vi "Shooter Code.vi"(10 "velocity_lower":dbl=1.0 format="%#_13g", 11 "velocity_upper":dbl=0.9 format="%#_13g") -> ()   [LabVIEW 2015]
panel:
  in  "index":dbl=1.0
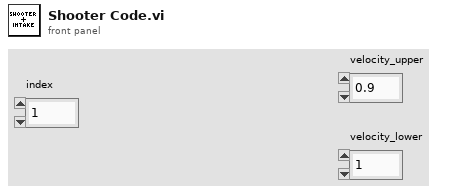
[diagram p1: front panel]
types:
  T1 = typedef "WPI_MotorControlDeviceRef.ctl" = cluster{"DeviceStatus":errorcluster, "Type":T2, "PWM":cluster{"PWM Channel":T3, "DeadBand":T4}, "CAN":cluster{"Device Number":u8, "Control Mode":T5, "Semaphore":T6, "Max Vout":dbl, "TalonSRX Control Mode":T7}, "Invert":bool}
  T2 = typedef "WPI_MotorControlType.ctl" = enum16{"PWM", "CAN", "CANTalonSRX"}
  T3 = typedef "FPGA_DIOPWMChannel.ctl" = enum8{"PWM 0", "PWM 1", "PWM 2", "PWM 3", "PWM 4", "PWM 5", "PWM 6", "PWM 7", "PWM 8", "PWM 9", "PWM MXP 0", "PWM MXP 1", "PWM MXP 2", "PWM MXP 3", "PWM MXP 4", "PWM MXP 5", "PWM MXP 6", "PWM MXP 7", "PWM MXP 8", "PWM MXP 9", "Invalid"}
  T4 = typedef "WPI_PWMDeadband.ctl" = cluster{"Name":string, "maxPositivePwm":i32, "minPositivePwm":i32, "centerPwm":i32, "maxNegativePwm":i32, "minNegativePwm":i32, "angularRange":u16}
  T5 = typedef "WPI_CANJaguar_ControlMode.ctl" = enum8{"Percent VBus", "Current", "Speed", "Position", "Voltage"}
  T6 = typedef "Semaphore RefNum" = refnum<k1>
  T7 = typedef "WPI_CANTalonSRX_APIControlMode.ctl" = enum8{"Percent VBus", "Speed", "Position", "Slave", "Unchanged / Invalid", "Voltage Compensation", "Current", "Motion Profile"}
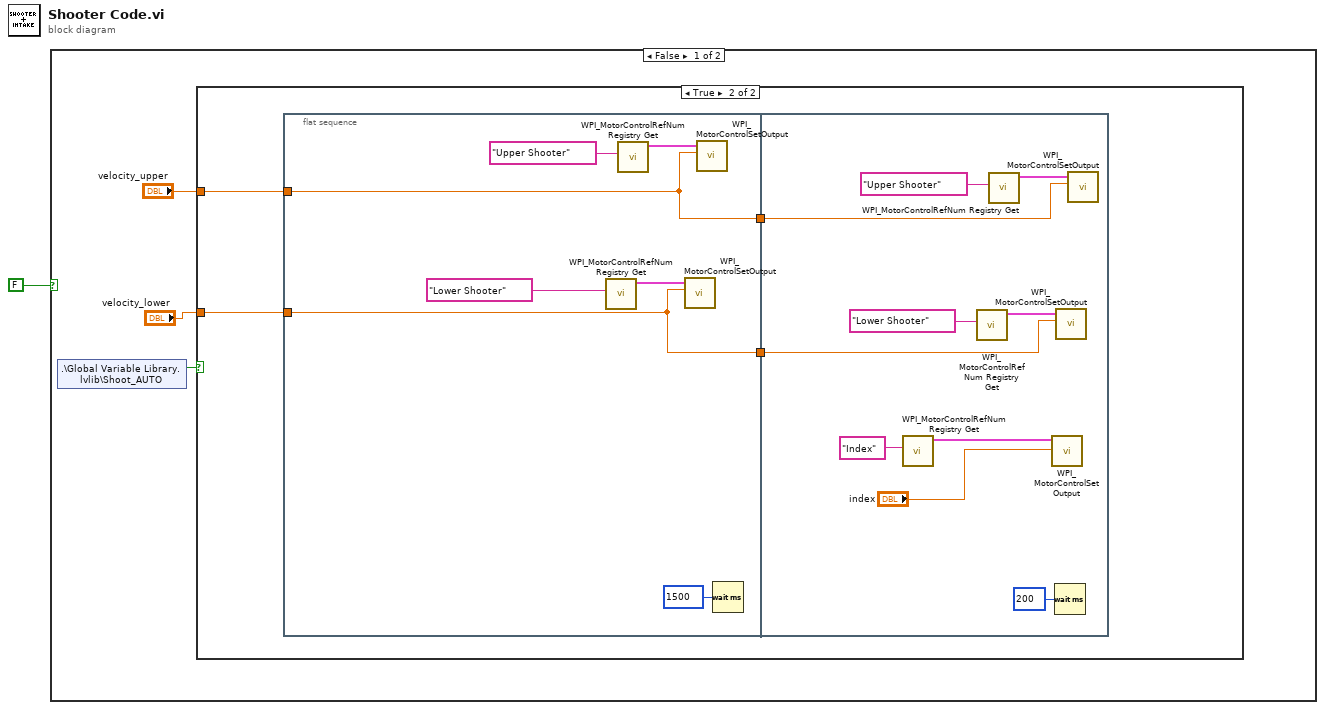
[diagram p0: block diagram]
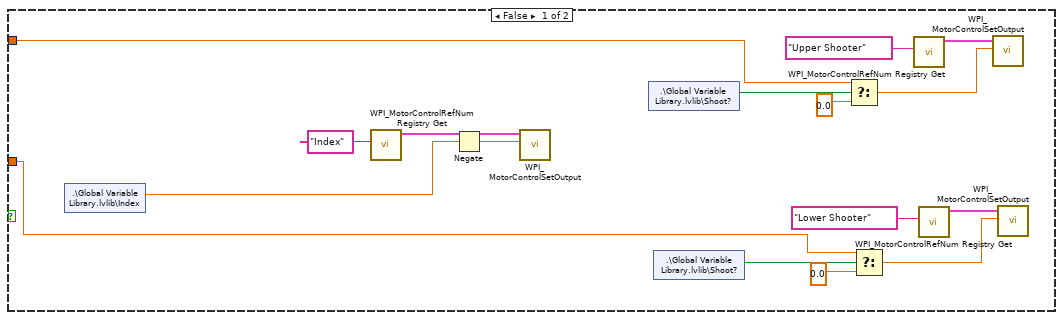
[diagram p2: hidden frame]
diagram:
  n1 = case shown="False" FALSE {
    frame False {
      n2 = shared-variable ".\\Global Variable Library.lvlib\\Shoot_AUTO"() -> (w4:bool)  [unwired: 1 in, 1 out]
      n3 = case shown="True" w4 {
        tunnel: "velocity_lower" -> [w5 w22]
        tunnel: "velocity_upper" -> [w6 w21]
        frame False {
          n4 = shared-variable ".\\Global Variable Library.lvlib\\Index"() -> (w7:dbl)  [unwired: 1 in, 1 out]
          n5 = call <vilib>:"WPI_MotorControlRefNum Registry Get.vi"("refnum name"="Index") -> ("MotorControlDevRef"=w10:T1)  [unwired: 9 in, 1 out]
          n6 = Negate(x=w7) -> (-x=w8:dbl)
          n7 = call <vilib>:"WPI_MotorControlSetOutput.vi"("Output"=w8, "MotorControlDevRef"=w10) -> ()  [unwired: 7 in, 3 out]
          n8 = shared-variable ".\\Global Variable Library.lvlib\\Shoot?"() -> (w18:bool)  [unwired: 1 in, 1 out]
          n9 = shared-variable ".\\Global Variable Library.lvlib\\Shoot?"() -> (w13:bool)  [unwired: 1 in, 1 out]
          n10 = Select(t=w6, s=w18, f=0.0) -> (s? t:f=w20:dbl)
          n11 = Select(t=w5, s=w13, f=0.0 ("f 2")) -> (s? t:f=w11:dbl)
          n12 = call <vilib>:"WPI_MotorControlRefNum Registry Get.vi"("refnum name"="Upper Shooter") -> ("MotorControlDevRef"=w16:T1)  [unwired: 9 in, 1 out]
          n13 = call <vilib>:"WPI_MotorControlRefNum Registry Get.vi"("refnum name"="Lower Shooter") -> ("MotorControlDevRef"=w15:T1)  [unwired: 9 in, 1 out]
          n14 = call <vilib>:"WPI_MotorControlSetOutput.vi"("Output"=w20, "MotorControlDevRef"=w16) -> ()  [unwired: 7 in, 3 out]
          n15 = call <vilib>:"WPI_MotorControlSetOutput.vi"("Output"=w11, "MotorControlDevRef"=w15) -> ()  [unwired: 7 in, 3 out]
        }
        frame True {
          n16 = flat-sequence {
            tunnel: [w27] -> w24
            tunnel: [w26] -> w23
            tunnel: w21 -> [w27]
            tunnel: w22 -> [w26]
            tunnel: w24 -> [w37]
            tunnel: w23 -> [w36]
            frame #0 {
              n17 = call <vilib>:"WPI_MotorControlRefNum Registry Get.vi"("refnum name"="Lower Shooter") -> ("MotorControlDevRef"=w30:T1)  [unwired: 9 in, 1 out]
              n18 = call <vilib>:"WPI_MotorControlRefNum Registry Get.vi"("refnum name"="Upper Shooter") -> ("MotorControlDevRef"=w29:T1)  [unwired: 9 in, 1 out]
              n19 = call <vilib>:"WPI_MotorControlSetOutput.vi"("Output"=w26, "MotorControlDevRef"=w30) -> ()  [unwired: 7 in, 3 out]
              n20 = call <vilib>:"WPI_MotorControlSetOutput.vi"("Output"=w27, "MotorControlDevRef"=w29) -> ()  [unwired: 7 in, 3 out]
              n21 = Wait (ms)(milliseconds to wait=u32 1500) -> ()  [unwired: 1 out]
            }
            frame #1 {
              n22 = call <vilib>:"WPI_MotorControlRefNum Registry Get.vi"("refnum name"="Index") -> ("MotorControlDevRef"=w34:T1)  [unwired: 9 in, 1 out]
              n23 = call <vilib>:"WPI_MotorControlRefNum Registry Get.vi"("refnum name"="Lower Shooter") -> ("MotorControlDevRef"=w39:T1)  [unwired: 9 in, 1 out]
              n24 = call <vilib>:"WPI_MotorControlRefNum Registry Get.vi"("refnum name"="Upper Shooter") -> ("MotorControlDevRef"=w40:T1)  [unwired: 9 in, 1 out]
              n25 = call <vilib>:"WPI_MotorControlSetOutput.vi"("Output"="index", "MotorControlDevRef"=w34) -> ()  [unwired: 7 in, 3 out]
              n26 = Wait (ms)(milliseconds to wait=u32 200) -> ()  [unwired: 1 out]
              n27 = call <vilib>:"WPI_MotorControlSetOutput.vi"("Output"=w36, "MotorControlDevRef"=w39) -> ()  [unwired: 7 in, 3 out]
              n28 = call <vilib>:"WPI_MotorControlSetOutput.vi"("Output"=w37, "MotorControlDevRef"=w40) -> ()  [unwired: 7 in, 3 out]
            }
          }
        }
      }
    }
    frame True {
    }
  }
